vi "Close Handle.vi"(8 "error in (no error)":errorcluster, 11 "Handle":i64) -> (0 "error out":errorcluster, 3 "Sucess?":bool)   [LabVIEW 2024, in "Power Requests.lvlib"]
uses:
  Power Requests.lvlib
  kernel32.dll
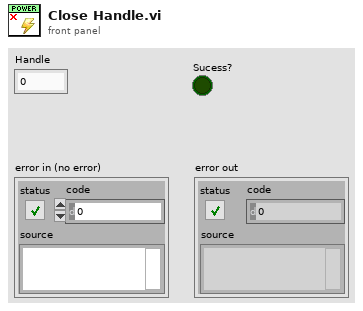
[diagram p1: front panel]
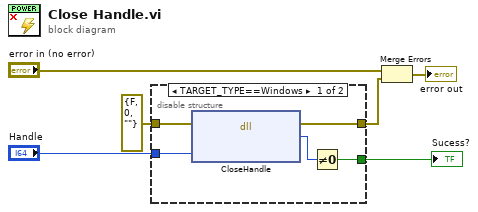
[diagram p0: block diagram]
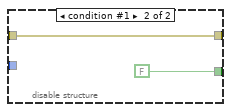
[diagram p2: hidden frame]
diagram:
  n1 = disable-structure shown="TARGET_TYPE==Windows" {
    disable-tunnel: [w11 w13] -> w2
    disable-tunnel: [w10 FALSE] -> w6
    disable-tunnel: errorcluster {"status"=FALSE, "code"=0, "source"=""} ("error in (no error)") -> [w9 w13]
    disable-tunnel: "Handle" -> [w7 _]
    frame condition #0 (active) {
      n2 = dll-call lib="kernel32.dll" fn="CloseHandle"(error in=w9, "_In_ HANDLE"=w7) -> (error out=w11:errorcluster, "BOOL"=w8:i32)  [unwired: 3 in, 1 out]
      n3 = Not Equal To 0?(x=w8) -> (x != 0?=w10:bool)
    }
    frame condition #1 {
    }
  }
  "Sucess?" <- w6
  n4 = Merge Errors("error in (no error)", w2) -> (→"error out":errorcluster)
